vi "ReadFromTermoDat.vi"() -> ()   [LabVIEW 2018]
uses:
  <vilib>/NI/Modbus Library/API/Wrapper/Create Serial Master.vi
  <vilib>/NI/Modbus Library/API/Master/Modbus Master.lvclass
  <vilib>/NI/Modbus Library/API/Wrapper/API Main.lvlib
panel:
  in  "serial type":enum16{"RTU", "ASCII"}(ring)
  in  "unit ID":u8=1
  out "register values":u16[](array[numeric])
  in  "stop":bool
  in  "baud rate":u32=9600
  in  "VISA resource name":refnum<visa-resource-name>
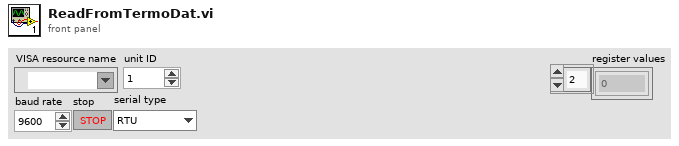
[diagram p1: front panel]
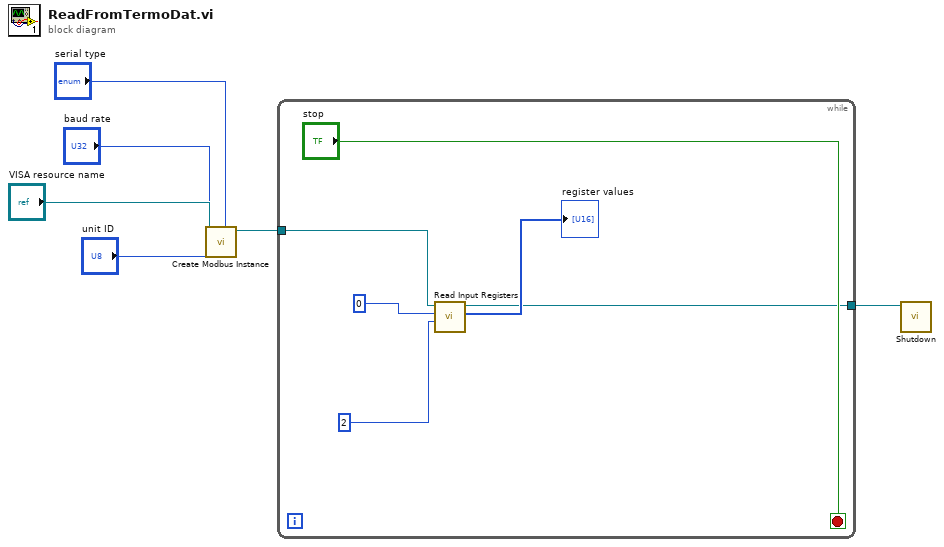
[diagram p0: block diagram]
diagram:
  n1 = call-poly <vilib>:"Create Modbus Instance.vi"("serial type"="serial type", "unit ID"="unit ID", "baud rate"="baud rate", "VISA resource name"="VISA resource name") -> ("serial master instance"=w4:refnum<class "Modbus Master.lvclass">)  [unwired: 6 in, 1 out]
  n2 = while {
    tunnel: w4 -> [w11]
    tunnel: [w8] -> w3
    stop <- "stop" stop-if-true
    n3 = call-dynamic "Read Input Registers.vi"("number of inputs"=u16 2, "starting address"=u16 0, "Modbus master in"=w11) -> ("register values"=→"register values":u16[], "Modbus master out"=w8:refnum<class "Modbus Master.lvclass">)  [unwired: 6 in, 1 out]
  }
  n4 = call-dynamic "Shutdown.vi"("Modbus master in"=w3) -> ()  [unwired: 10 in, 1 out]
